vi "WS1021 MEMS Only 24DUT CV Sweep Header BA.vi"(8 "Error In":errorcluster) -> (0 "Error Out":errorcluster, 3 "Name Calculated Header":string[](array[string]))   [LabVIEW 2017]
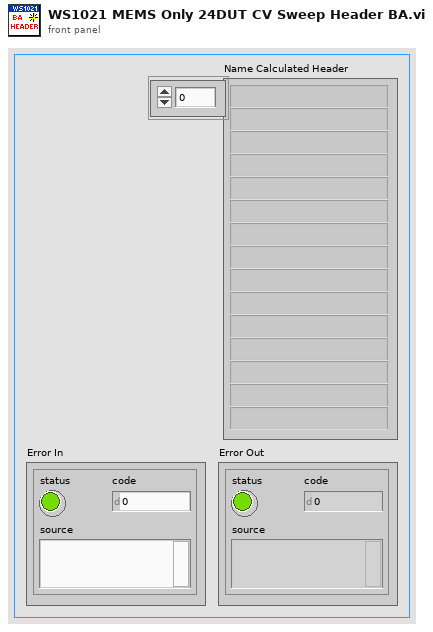
[diagram p1: front panel]
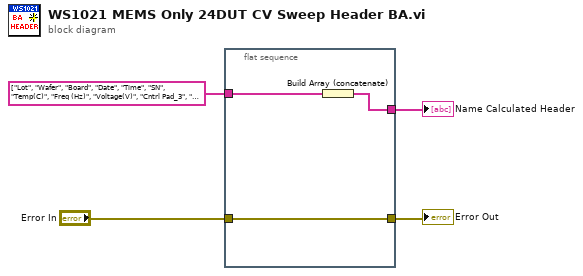
[diagram p0: block diagram]
diagram:
  n1 = flat-sequence {
    tunnel: "Error In" -> [w7]
    tunnel: [w7] -> w4
    tunnel: string[] ["Lot", "Wafer", "Board", "Date", "Time", "SN", "Temp(C)", "Freq (Hz)", "Voltage(V)", "Cntrl Pad_3", "C1 (fF)", "Cntrl Pad_1", "C3 (fF)", "Cntrl Pad_5", "C4 (fF)", "Cntrl Pad_4", "C2 (fF)", "Cntrl Pad_2", "C5 (fF)", "Cntrl Pad_6", "C6 (fF)", "C1_DCap (fF)", "C3_DCap (fF)", "C4_DCap (fF)", "C2_DCap (fF)", "C5_DCap (fF)", "C6_DCap (fF)", "Command", "Test Program"] -> [w6]
    tunnel: [w5] -> w2
    frame #0 {
      n2 = Build Array (concatenate)(w6) -> (w5:string[])
    }
  }
  "Name Calculated Header" <- w2
  "Error Out" <- w4
